vi "Vac_lim.vi"(10 "IN Vdc":dbl=750.0) -> (2 "OUT Vdc":dbl)   [LabVIEW 2021]
panel:
  out "?":bool
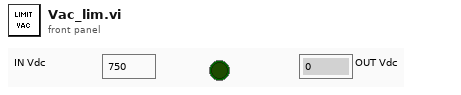
[diagram p1: front panel]
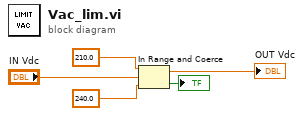
[diagram p0: block diagram]
diagram:
  n1 = In Range and Coerce(upper limit=210.0 ("x"), x="IN Vdc", lower limit=240.0 ("x")) -> (coerced(x)=→"OUT Vdc":dbl, In Range?=→"?":bool)
